vi "set_user_comments.vi"(8 "error in (no error)":errorcluster, 10 "details source":string, 11 "ErrorController in":refnum<class "ErrorController.lvclass">) -> (0 "error out":errorcluster, 3 "ErrorController out":refnum<class "ErrorController.lvclass">)   [LabVIEW 2010, in "ErrorController.lvclass"]
uses:
  ErrorController.lvclass
panel:
  in  "button:details":bool
  in  "configuring":bool
  in  "comments":string caption="Further comments:"
  in  "button: ok":bool
  in  "new error":bool
  in  "click pattern text":string
  in  "details text":string
  in  "details":bool
  in  "single sweep":bool
  in  "click pattern":bool
  in  "pressed buttons":bool
  in  "nothing":bool
  # "What happened?"
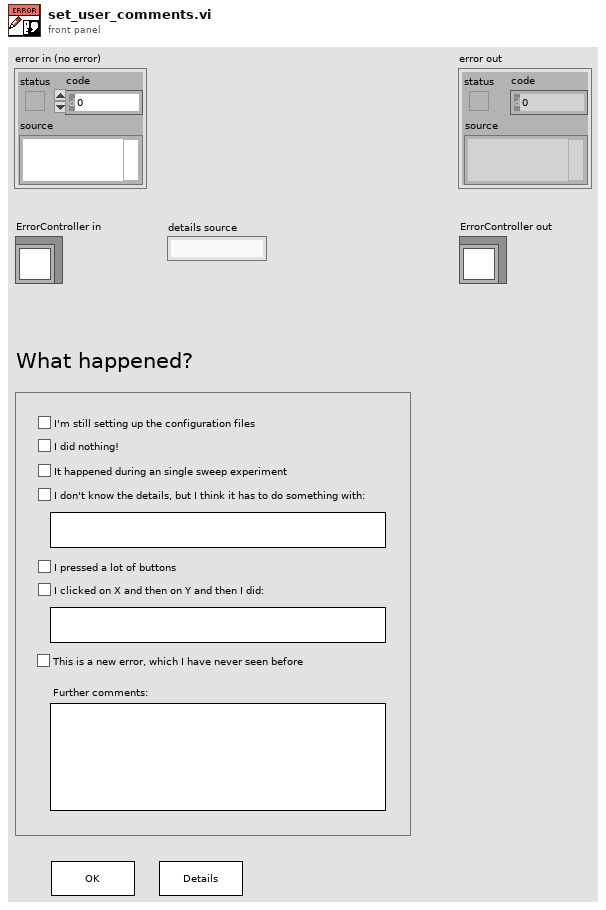
[diagram p1: front panel]
types:
  T1 = enum8{"Enabled", "Disabled", "Disabled and Grayed Out"}
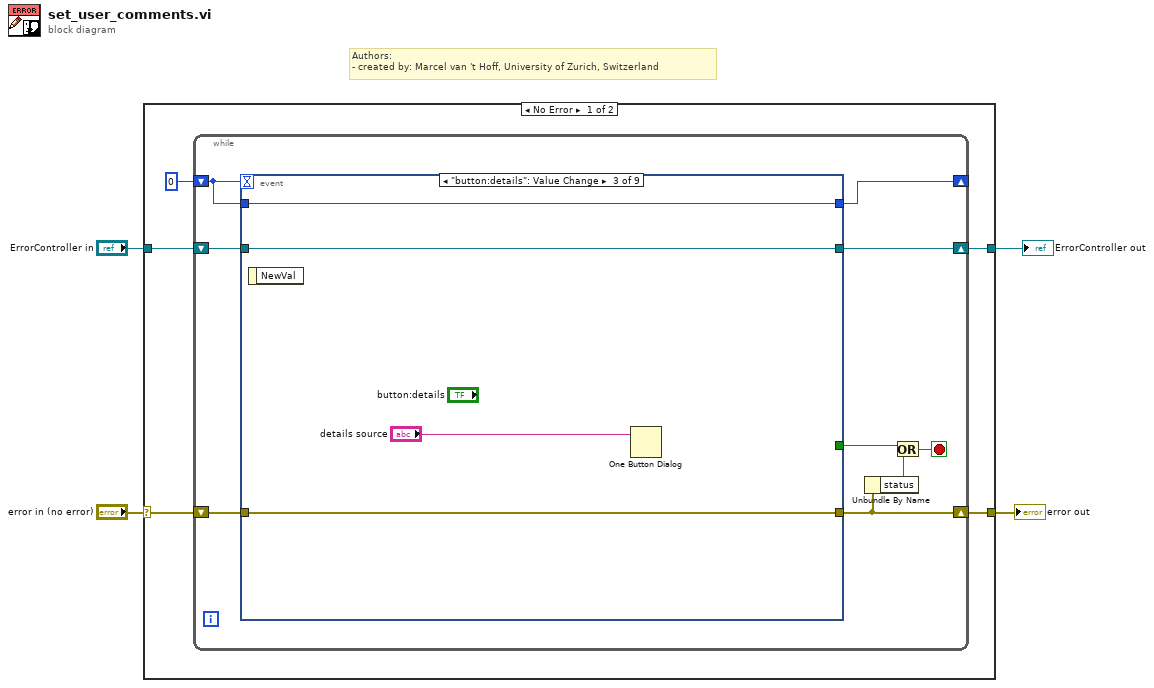
[diagram p0: block diagram]
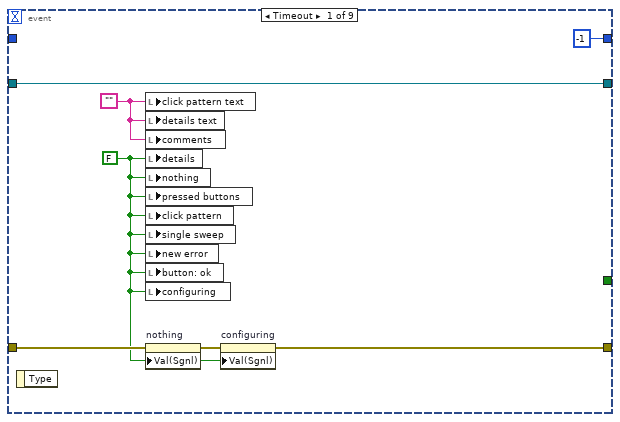
[diagram p2: hidden frame]
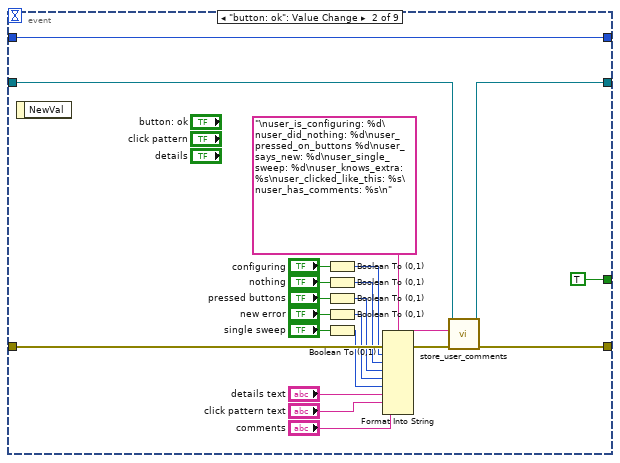
[diagram p3: hidden frame]
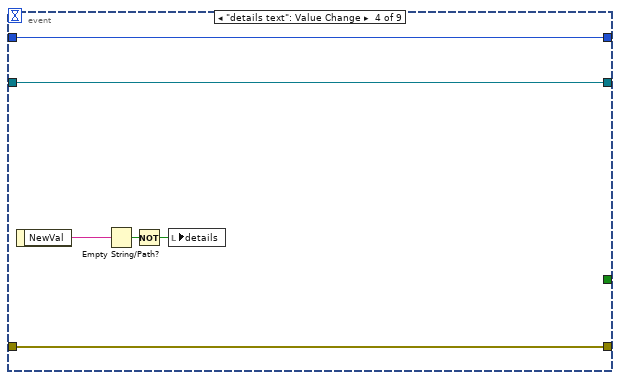
[diagram p4: hidden frame]
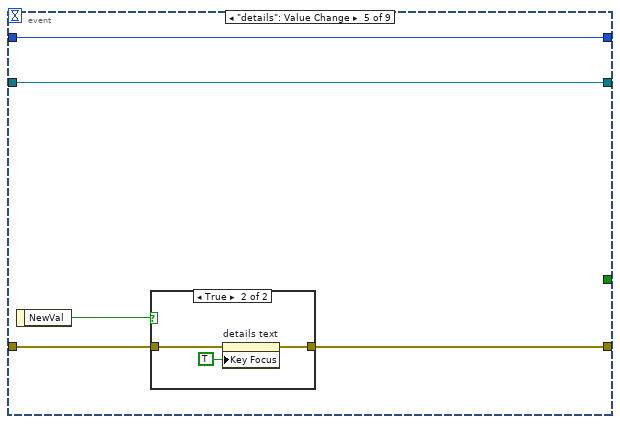
[diagram p5: hidden frame]
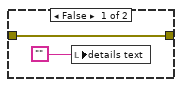
[diagram p6: hidden frame]
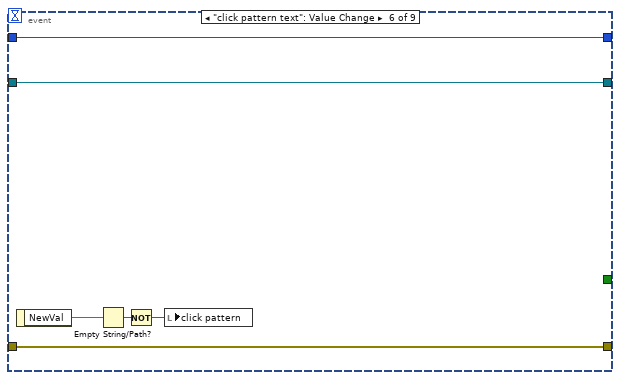
[diagram p7: hidden frame]
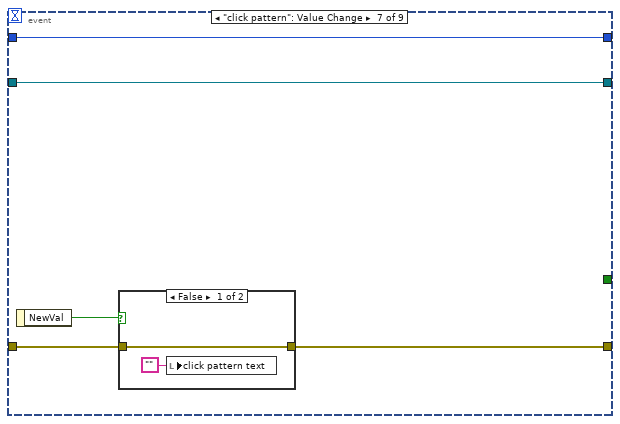
[diagram p8: hidden frame]
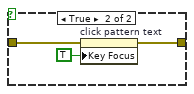
[diagram p9: hidden frame]
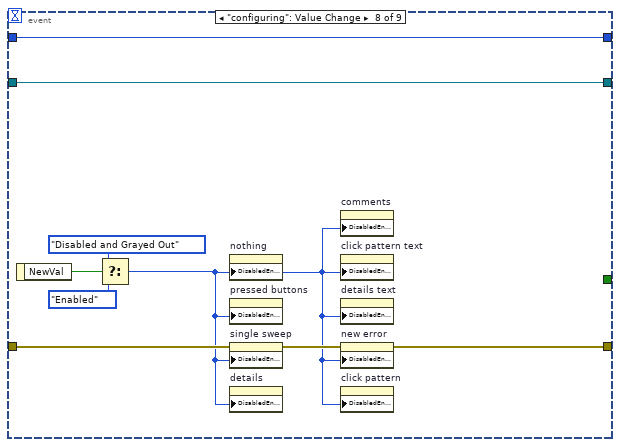
[diagram p10: hidden frame]
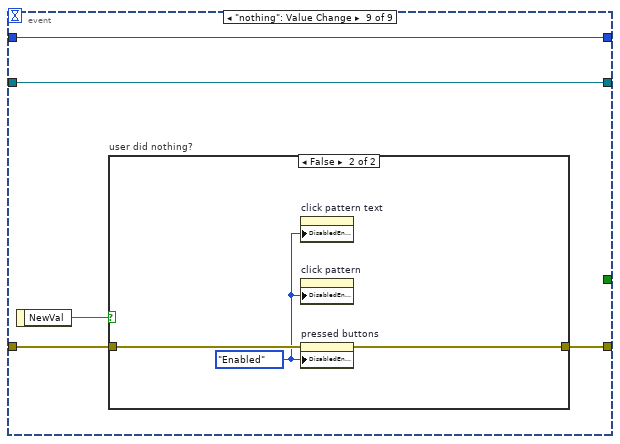
[diagram p11: hidden frame]
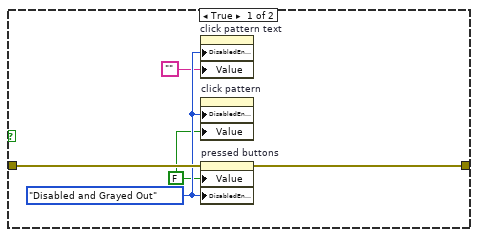
[diagram p12: hidden frame]
diagram:
  # "Authors: \n- created by: Marcel van 't Hoff, University of Zurich, Switzerland"
  n1 = case shown="No Error" "error in (no error)" {
    selector: "error in (no error)" -> [w8 w107]
    tunnel: [w9 w107] -> w3
    tunnel: [w7 w106] -> w1
    tunnel: "ErrorController in" -> [w6 w106]
    frame No Error {
      n2 = while {
        shift-right: [w15] -> w9
        shift-left: w8 -> [w18]
        shift-right: [w17] -> w7
        shift-left: w6 -> [w16]
        shift-right: [w10] -> _
        shift-left: 0 -> [w11]
        stop <- w12 stop-if-true
        n3 = event shown="[2] \"button:details\": Value Change" {
          selector: _ -> [_ _ _ _ _ _ _ _ _]
          dyn-events: _ -> [_ _ _ _ _ _ _ _ _]
          timeout: w11 -> [_ _ _ _ _ _ _ _ _]
          tunnel: [w20 w28 w48 w53 w59 w69 w76 w85 w94] -> w15
          tunnel: w18 -> [w22 w45 w48 w53 w60 w69 w77 w87 w95]
          tunnel: [w25 w26 w51 w57 w62 w73 w78 w92 w97] -> w17
          tunnel: w16 -> [w25 w27 w51 w57 w62 w73 w78 w92 w97]
          tunnel: [_ TRUE _ _ _ _ _ _ _] -> w13
          tunnel: [-1 w46 w50 w52 w58 w68 w74 w91 w96] -> w10
          tunnel: w11 -> [_ w46 w50 w52 w58 w68 w74 w91 w96]
          event Timeout {
            w19 = FALSE
            w23 = ""
            n4 = event-data() -> ()  [unwired: 1 in, 1 out]
            n5 = local write "click pattern text"(w23) -> ()
            n6 = local write "details text"(w23) -> ()
            n7 = local write "comments"(w23) -> ()
            n8 = local write "details"(w19) -> ()
            n9 = local write "nothing"(w19) -> ()
            n10 = local write "pressed buttons"(w19) -> ()
            n11 = local write "click pattern"(w19) -> ()
            n12 = local write "single sweep"(w19) -> ()
            n13 = local write "new error"(w19) -> ()
            n14 = local write "button: ok"(w19) -> ()
            n15 = local write "configuring"(w19) -> ()
            n16 = property on="nothing" class="Bool (strict)"(error in=w22, "Val(Sgnl)"=w19) -> (error out=w21:errorcluster)  [unwired: 1 in, 1 out]
            n17 = property on="configuring" class="Bool (strict)"(error in=w21, "Val(Sgnl)"=w19) -> (error out=w20:errorcluster)  [unwired: 1 in, 1 out]
          }
          event "button: ok": Value Change {
            n18 = event-data() -> ()  [unwired: 1 in, 1 out]
            n19 = Boolean To (0,1)(Boolean="configuring") -> (0, 1=w32:i16)
            n20 = Boolean To (0,1)(Boolean="nothing") -> (0, 1=w33:i16)
            n21 = Boolean To (0,1)(Boolean="pressed buttons") -> (0, 1=w34:i16)
            n22 = Boolean To (0,1)(Boolean="new error") -> (0, 1=w35:i16)
            n23 = Boolean To (0,1)(Boolean="single sweep") -> (0, 1=w36:i16)
            n24 = Format Into String(format string="\nuser_is_configuring: %d\nuser_did_nothing: %d\nuser_pressed_on_buttons %d\nuser_says_new: %d\nuser_single_sweep: %d\nuser_knows_extra: %s\nuser_clicked_like_this: %s\nuser_has_comments: %s\n", error in=w45, w32, w33, w34, w35, w36, "details text", "click pattern text", "comments") -> (resulting string=w30:string, error out=w29:errorcluster)  [unwired: 1 in]
            n25 = call-dynamic "store_user_comments.vi"("error in (no error)"=w29, "user comments in"=w30, "ErrorController in"=w27) -> ("error out"=w28:errorcluster, "ErrorController out"=w26:refnum<class "ErrorController.lvclass">)  [unwired: 7 in]
          }
          event "button:details": Value Change {
            n26 = event-data() -> ()  [unwired: 1 in, 1 out]
            n27 = One Button Dialog(message="details source") -> ()  [unwired: 1 in, 1 out]
          }
          event "details text": Value Change {
            n28 = event-data() -> ("NewVal"=w56:string)  [unwired: 1 in]
            n29 = Empty String/Path?(string/path=w56) -> (empty?=w55:bool)
            n30 = Not(x=w55) -> (.not. x?=w54:bool)
            n31 = local write "details"(w54) -> ()
          }
          event "details": Value Change {
            n32 = event-data() -> ("NewVal"=w61:bool)  [unwired: 1 in]
            n33 = case shown="True" w61 {
              tunnel: w60 -> [w64 w67]
              tunnel: [w64 w65] -> w59
              frame False {
                n34 = local write "details text"("") -> ()
              }
              frame True {
                n35 = property on="details text" class="Str"(error in=w67, "Key Focus"=TRUE) -> (error out=w65:errorcluster)  [unwired: 1 in, 1 out]
              }
            }
          }
          event "click pattern text": Value Change {
            n36 = event-data() -> ("NewVal"=w71:string)  [unwired: 1 in]
            n37 = Empty String/Path?(string/path=w71) -> (empty?=w72:bool)
            n38 = Not(x=w72) -> (.not. x?=w70:bool)
            n39 = local write "click pattern"(w70) -> ()
          }
          event "click pattern": Value Change {
            n40 = event-data() -> ("NewVal"=w75:bool)  [unwired: 1 in]
            n41 = case shown="False" w75 {
              tunnel: w77 -> [w80 w83]
              tunnel: [w80 w81] -> w76
              frame False {
                n42 = local write "click pattern text"("") -> ()
              }
              frame True {
                n43 = property on="click pattern text" class="Str"(error in=w83, "Key Focus"=TRUE) -> (error out=w81:errorcluster)  [unwired: 1 in, 1 out]
              }
            }
          }
          event "configuring": Value Change {
            n44 = event-data() -> ("NewVal"=w90:bool)  [unwired: 1 in]
            n45 = Select(t=T1."Disabled and Grayed Out" ("Disabled"), s=w90, f=T1."Enabled" ("Disabled")) -> (s? t:f=w84:T1)
            n46 = property on="nothing" class="Bool (strict)"("DisabledEnum"=w84) -> ()  [unwired: 2 in, 2 out]
            n47 = property on="pressed buttons" class="Bool (strict)"("DisabledEnum"=w84) -> ()  [unwired: 2 in, 2 out]
            n48 = property on="single sweep" class="Bool (strict)"(error in=w87, "DisabledEnum"=w84) -> (error out=w86:errorcluster)  [unwired: 1 in, 1 out]
            n49 = property on="details" class="Bool (strict)"("DisabledEnum"=w84) -> ()  [unwired: 2 in, 2 out]
            n50 = property on="comments" class="Str"("DisabledEnum"=w84) -> ()  [unwired: 2 in, 2 out]
            n51 = property on="click pattern text" class="Str"("DisabledEnum"=w84) -> ()  [unwired: 2 in, 2 out]
            n52 = property on="details text" class="Str"("DisabledEnum"=w84) -> ()  [unwired: 2 in, 2 out]
            n53 = property on="new error" class="Bool (strict)"(error in=w86, "DisabledEnum"=w84) -> (error out=w85:errorcluster)  [unwired: 1 in, 1 out]
            n54 = property on="click pattern" class="Bool (strict)"("DisabledEnum"=w84) -> ()  [unwired: 2 in, 2 out]
          }
          event "nothing": Value Change {
            n55 = event-data() -> ("NewVal"=w93:bool)  [unwired: 1 in]
            n56 = case "user did nothing?" shown="False" w93 {
              tunnel: w95 -> [w102 w105]
              tunnel: [w101 w104] -> w94
              frame True {
                w100 = T1."Disabled and Grayed Out" ("Disabled")
                w99 = FALSE ("pressed buttons")
                n57 = property on="click pattern text" class="Str"("DisabledEnum"=w100, "Value"="") -> ()  [unwired: 2 in, 2 out]
                n58 = property on="click pattern" class="Bool (strict)"("DisabledEnum"=w100, "Value"=w99) -> ()  [unwired: 2 in, 2 out]
                n59 = property on="pressed buttons" class="Bool (strict)"(error in=w102, "Value"=w99, "DisabledEnum"=w100) -> (error out=w101:errorcluster)  [unwired: 1 in, 1 out]
              }
              frame False {
                w103 = T1."Enabled" ("Disabled")
                n60 = property on="click pattern text" class="Str"("DisabledEnum"=w103) -> ()  [unwired: 2 in, 2 out]
                n61 = property on="click pattern" class="Bool (strict)"("DisabledEnum"=w103) -> ()  [unwired: 2 in, 2 out]
                n62 = property on="pressed buttons" class="Bool (strict)"(error in=w105, "DisabledEnum"=w103) -> (error out=w104:errorcluster)  [unwired: 1 in, 1 out]
              }
            }
          }
        }
        n63 = Unbundle By Name(w15) -> ("status"=w14:bool)
        n64 = Or(x=w13, y=w14) -> (x .or. y?=w12:bool)
      }
    }
    frame Error {
    }
  }
  "error out" <- w3
  "ErrorController out" <- w1
